vi "Get Standard VI Data.vi"(8 "error in (no error)":errorcluster, 11 "VI in":refnum<vi>) -> (0 "error out":errorcluster, 2 "VI Properties":T1, 3 "VI out":refnum<vi>)   [LabVIEW 2023, in "VI Properties Editor.lvlib"]
doc: "Gets all data for a standard VI."
uses:
  VI Properties Editor.lvlib
  CTLs/VI Properties.ctl
  <vilib>/picture/picture.llb/imagedata.ctl
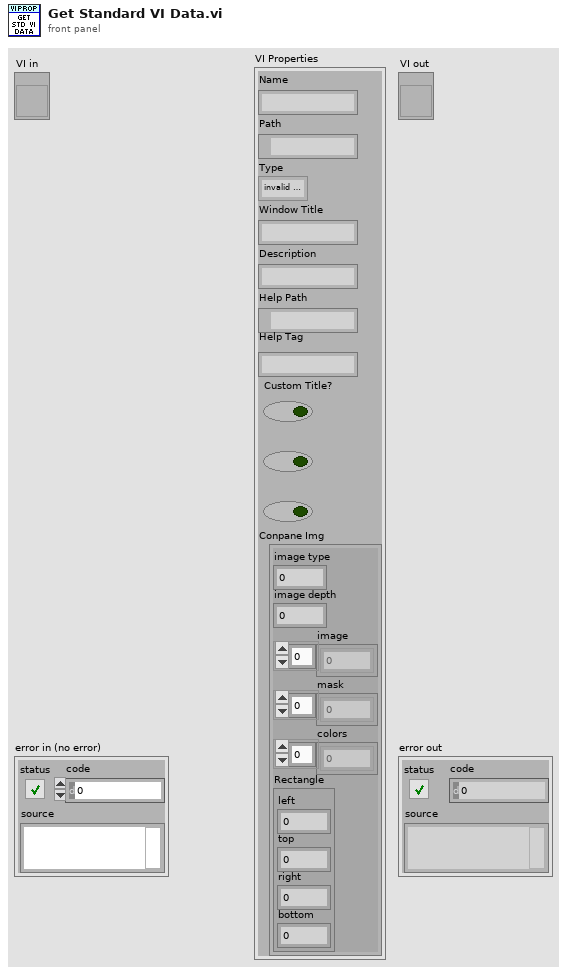
[diagram p1: front panel]
types:
  T1 = typedef "VI Properties Editor.lvlib/VI Properties.ctl" = cluster{"Name":string, "Path":path, "Type":enum32{"invalid VI type", "Standard VI", "Control VI", "Global VI", "Polymorphic VI", "Configuration VI", "SubSystem", "Facade VI", "Method VI", "Statechart Diagram VI"}, "Window Title":string, "Description":string, "Help Path":path, "Help Tag":string, "Custom Title?":bool, "Reentrant?":bool, "Inlined?":bool, "Conpane Img":T2}
  T2 = typedef "imagedata.ctl" = cluster{"image type":i32, "image depth":i32, "image":u8[], "mask":u8[], "colors":u32[], "Rectangle":cluster{"left":i16, "top":i16, "right":i16, "bottom":i16}}
  T3 = enum32{"invalid VI type", "Standard VI", "Control VI", "Global VI", "Polymorphic VI", "Configuration VI", "SubSystem", "Facade VI", "Method VI", "Statechart Diagram VI"}
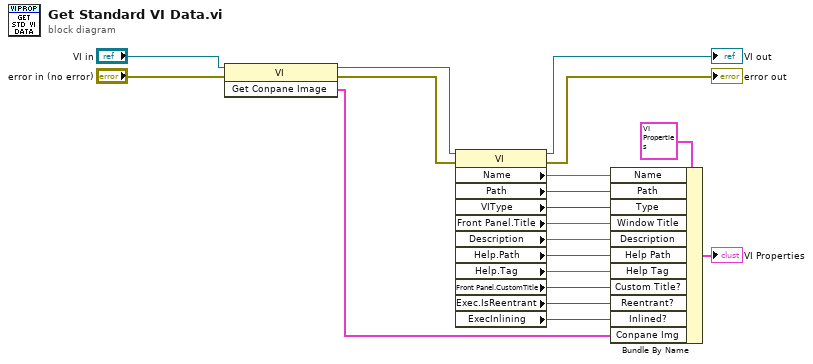
[diagram p0: block diagram]
diagram:
  n1 = invoke class="VI" method="Get Conpane Image"(reference="VI in", error in="error in (no error)") -> (reference out=w7:refnum<vi>, error out=w6:errorcluster, "Get Conpane Image"=w9:T2)  [unwired: 1 in]
  n2 = property class="VI"(reference=w7, error in=w6) -> (reference out=→"VI out":refnum<vi>, error out=→"error out":errorcluster, "Name"=w18:string, "Path"=w17:path, "VIType"=w16:T3, "Front Panel.Title"=w2:string, "Description"=w15:string, "Help.Path"=w14:path, "Help.Tag"=w13:string, "Front Panel.CustomTitle"=w1:bool, "Exec.IsReentrant"=w12:bool, "ExecInlining"=w11:bool)
  n3 = Bundle By Name(cluster=T1 {"Name"="", "Path"=path "", "Type"=enum."invalid VI type", "Window Title"="", "Description"="", "Help Path"=path "", "Help Tag"="", "Custom Title?"=FALSE, "Reentrant?"=FALSE, "Inlined?"=FALSE, "Conpane Img"={"image type"=0, "image depth"=0, "image"=[], "mask"=[], "colors"=[], "Rectangle"={"left"=0, "top"=0, "right"=0, "bottom"=0}}} ("VI Properties"), "Name"=w18, "Path"=w17, "Type"=w16, "Window Title"=w2, "Description"=w15, "Help Path"=w14, "Help Tag"=w13, "Custom Title?"=w1, "Reentrant?"=w12, "Inlined?"=w11, "Conpane Img"=w9) -> (→"VI Properties":T1)
